vi "WriteEvtRptArrayRequest.vi"(8 "error in (no error)":errorcluster, 10 "EvtRptArray":T1[](array[typedef]) {"Synx" format="%#_4g"}, 11 "ModuleID":i32) -> (0 "error out":errorcluster)   [LabVIEW 2017, in "OutputToFileModule.lvlib"]
uses:
  OutputToFileModule.lvlib
  EventPlugins/EventPluginBaseClass/TypeDefs/clEvtReport.ctl
  Private/clEventType.ctl
  <vilib>/Utility/error.llb/Error Cluster From Error Code.vi
  <vilib>/ErrorRing/Error Ring.xnode
  EventPlugins/EventPluginBaseClass/EventPluginBaseClass.lvclass
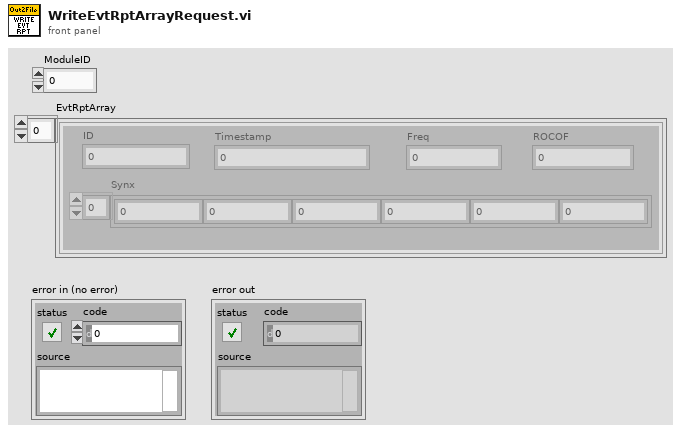
[diagram p1: front panel]
types:
  T1 = typedef "EventPlugins.lvlib/EventPluginBaseClass.lvclass/clEvtReport.ctl" = cluster{"Timestamp":dbl, "Synx":cdb[], "Freq":dbl, "ROCOF":dbl, "ID":i16}
  T2 = typedef "OutputToFileModule.lvlib/clRequestEvents.ctl" = cluster{"StopRequest":refnum<user-event>, "LoadPluginRequest":refnum<user-event>, "ReadPathToPluginRequest":refnum<user-event>, "WriteEvtRptRequest":refnum<user-event>, "WritePmuImpairRptRequest":refnum<user-event>, "WriteNetTimeRequest":refnum<user-event>, "WritePktLossRequest":refnum<user-event>, "WritePmuConfigRequest":refnum<user-event>, "ReadPmuConfigRequest":refnum<user-event>, "WriteOutPathRequest":refnum<user-event>, "ReadOutPathRequest":refnum<user-event>, "WriteFlagImpairRequest":refnum<user-event>, "OutputRefFileRequest":refnum<user-event>, "OutputImpairedFileRequest":refnum<user-event>, "OutputErrorDataRequest":refnum<user-event>, "OpenConfigRequest":refnum<user-event>, "ShowPanel":refnum<user-event>}
  T3 = typedef "OutputToFileModule.lvlib/clEventType.ctl" = cluster{"ModuleID":i32, "Data":variant}
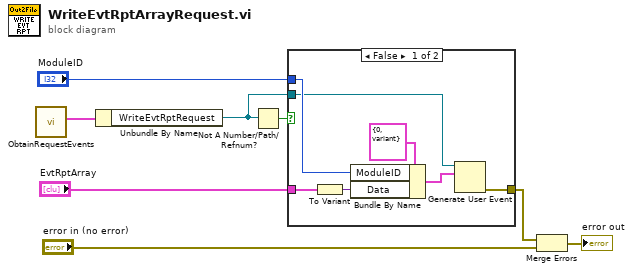
[diagram p0: block diagram]
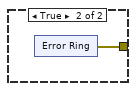
[diagram p2: hidden frame]
diagram:
  n1 = call "ObtainRequestEvents.vi"() -> ("clRequestEvents"=w8:T2)  [unwired: 10 in, 1 out]
  n2 = Unbundle By Name(w8) -> ("WriteEvtRptRequest"=w5:refnum<user-event>)
  n3 = Not A Number/Path/Refnum?(number/path/refnum=w5) -> (NaN/Path/Refnum?=w7:bool)
  n4 = case shown="False" w7 {
    tunnel: "ModuleID" -> [w14 _]
    tunnel: w5 -> [w13 _]
    tunnel: [w11 w16] -> w4
    tunnel: "EvtRptArray" -> [w9 _]
    frame False {
      n5 = To Variant(anything=w9) -> (Variant=w10:variant)
      n6 = Bundle By Name(cluster=T3 {"ModuleID"=0, "Data"=variant} ("clEventType"), "ModuleID"=w14, "Data"=w10) -> (w12:T3)
      n7 = Generate User Event(user event=w13, event data cluster=w12) -> (error out=w11:errorcluster)  [unwired: 2 in, 1 out]
    }
    frame True {
      n8 = xnode "Error Ring"() -> ("error out"=w16:errorcluster)
    }
  }
  n9 = Merge Errors(w4, "error in (no error)") -> (→"error out":errorcluster)
